vi "Set field (linear and oscillate).vi"(6 "Rate(Oe/s)":dbl, 7 "semaphore":T1 caption="信号量", 8 "error in":errorcluster, 9 "数值":dbl format="%#_13g", 10 "Approach":enum16{"Linear", "Oscillate"}(ring)=enum."Oscillate", 11 "VISA Resource Name":refnum<visa-resource-name>) -> (0 "error out 2":errorcluster caption="error out", 2 "Oscillate?":bool, 3 "dup VISA session":refnum<visa-resource-name>, 5 "semaphore out":T1 caption="信号量输出")   [LabVIEW 2019, in "9T cmag.lvlib"]
uses:
  9T cmag.lvlib
  SubVI.lvlib
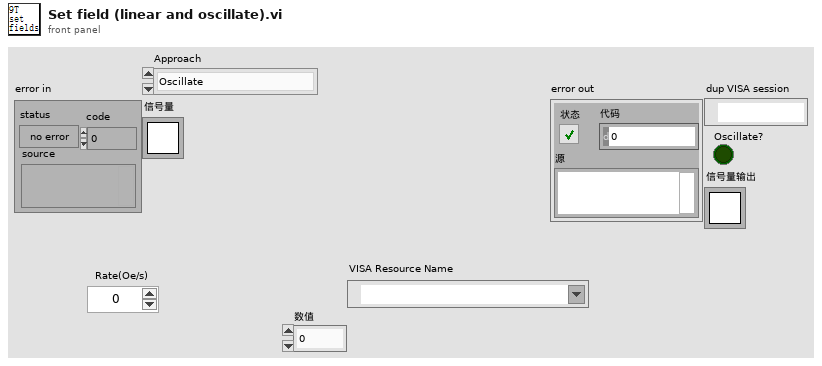
[diagram p1: front panel]
types:
  T1 = typedef "Semaphore RefNum" = refnum<k1>
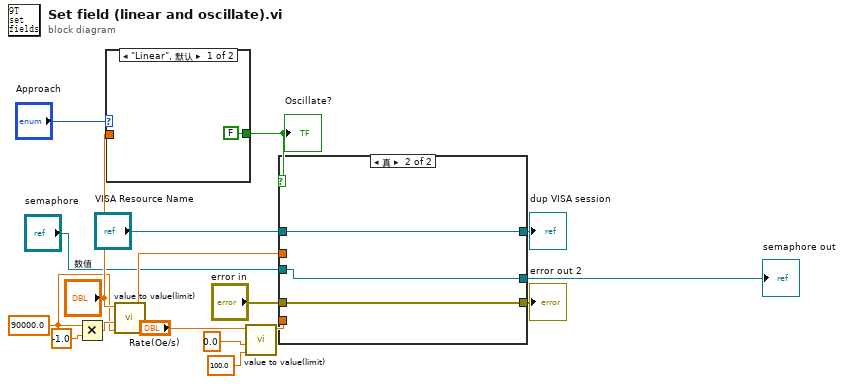
[diagram p0: block diagram]
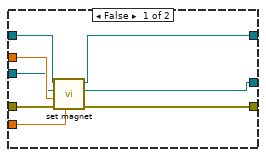
[diagram p2: hidden frame]
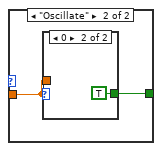
[diagram p3: hidden frame]
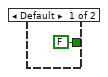
[diagram p4: hidden frame]
diagram:
  w3 = 90000.0 ("x")
  n1 = Multiply(x=w3, y=-1.0) -> (x*y=w6:dbl)
  n2 = case shown="\"Linear\", 默认" "Approach" {
    tunnel: "数值" -> [_ w20]
    tunnel: [FALSE w19] -> w17
    frame "Linear", Default {
    }
    frame "Oscillate" {
      n3 = case shown="0" w20 {
        tunnel: w20 -> [_ _]
        tunnel: [FALSE TRUE] -> w19
        frame Default {
        }
        frame 0 {
        }
      }
    }
  }
  "Oscillate?" <- w17
  n4 = call "value to value(limit).vi"("high limit"=w3, "low limit"=w6, "数值 in"="数值") -> ("数值 out"=w4:dbl)  [unwired: 8 in]
  n5 = call "value to value(limit).vi"("high limit"=100.0 ("y"), "low limit"=0.0, "数值 in"="Rate(Oe/s)") -> ("数值 out"=w8:dbl)  [unwired: 8 in]
  n6 = case shown="真" w17 {
    tunnel: "VISA Resource Name" -> [w30 w33]
    tunnel: w4 -> [w29 _]
    tunnel: "error in" -> [w27 w32]
    tunnel: [w28 w33] -> w13
    tunnel: [w26 w32] -> w14
    tunnel: w8 -> [w25 _]
    tunnel: [w24 w31] -> w2
    tunnel: "semaphore" -> [w23 w31]
    frame False {
      n7 = call "set magnet.vi"("Rate(Oe/s)"=w25, "error in (no error)"=w27, "Magnet field(Oe)"=w29, "semaphore"=w23, "VISA Resource Name"=w30) -> ("error out"=w26:errorcluster, "semaphore out"=w24:T1, "dup VISA session"=w28:refnum<visa-resource-name>)  [unwired: 4 in]
    }
    frame True {
    }
  }
  "error out 2" <- w14
  "dup VISA session" <- w13
  "semaphore out" <- w2
